vi "WriteHSpeed.vi"(8 "error in":errorcluster, 9 "Reply length":i32=-1, 10 "write buffer":string, 11 "VISA Refnum in":refnum<visa-resource-name>) -> (0 "error out":errorcluster, 2 "read buffer":string, 3 "VISA Refnum out":refnum<visa-resource-name>)   [LabVIEW 2020]
panel:
  out "buffer":u32
  out "Bytes at Port":u32
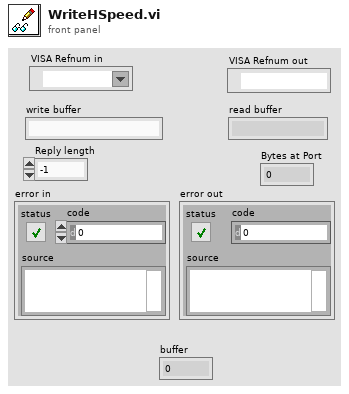
[diagram p1: front panel]
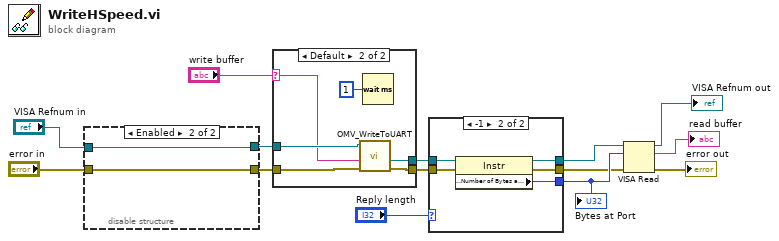
[diagram p0: block diagram]
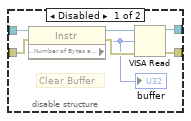
[diagram p2: hidden frame]
diagram:
  n1 = disable-structure shown="Enabled" {
    disable-tunnel: "error in" -> [w18 w22]
    disable-tunnel: [w17 w22] -> w3
    disable-tunnel: "VISA Refnum in" -> [w16 w23]
    disable-tunnel: [w15 w23] -> w1
    frame Disabled {
      # "Clear Buffer"
      n2 = property class="Instr"(reference=w16, error in=w18) -> (reference out=w19:refnum<visa-resource-name>, error out=w21:errorcluster, "Serial Settings:Number of Bytes at Serial Port"=w20:u32)
      "buffer" <- w20
      n3 = VISA Read(VISA resource name=w19, byte count=w20, error in (no error)=w21) -> (VISA resource name out=w15:refnum<visa-resource-name>, error out=w17:errorcluster)  [unwired: 2 out]
    }
    frame Enabled {
    }
  }
  n4 = case shown="Default" "write buffer" {
    selector: "write buffer" -> [_ w26]
    tunnel: w1 -> [w25 w30]
    tunnel: w3 -> [w24 w29]
    tunnel: [w25 w27] -> w12
    tunnel: [w24 w28] -> w11
    frame "" {
    }
    frame Default {
      n5 = call "OMV_WriteToUART.vi"("error in"=w29, "Text to write"=w26, "VISA resource name"=w30) -> ("error out"=w28:errorcluster, "VISA Refnum out"=w27:refnum<visa-resource-name>)  [unwired: 7 in]
      n6 = Wait (ms)(milliseconds to wait=u32 1) -> ()  [unwired: 1 out]
    }
  }
  n7 = case shown="-1" "Reply length" {
    selector: "Reply length" -> [w32 _]
    tunnel: [w34 w39] -> w14
    tunnel: [w32 w38] -> w13
    tunnel: w12 -> [w34 w37]
    tunnel: w11 -> [w33 w36]
    tunnel: [w33 w35] -> w9
    frame Default {
    }
    frame -1 {
      n8 = property class="Instr"(reference=w37, error in=w36) -> (reference out=w39:refnum<visa-resource-name>, error out=w35:errorcluster, "Serial Settings:Number of Bytes at Serial Port"=w38:u32)
    }
  }
  "Bytes at Port" <- w13
  n9 = VISA Read(VISA resource name=w14, byte count=w13, error in (no error)=w9) -> (VISA resource name out=→"VISA Refnum out":refnum<visa-resource-name>, read buffer=→"read buffer":string, error out=→"error out":errorcluster)  [unwired: 1 out]
